vi "打开电脑摄像头获取图像.vi"() -> ()   [LabVIEW 2014]
uses:
  <vilib>/userdefined/High Color/IMAQdx.ctl
  <vilib>/vision/driver/NI_Vision_Acquisition_Software.lvlib
panel:
  out "Session Out":T1
  out "Image Out":T2(plugin-control)
  in  "停止":bool
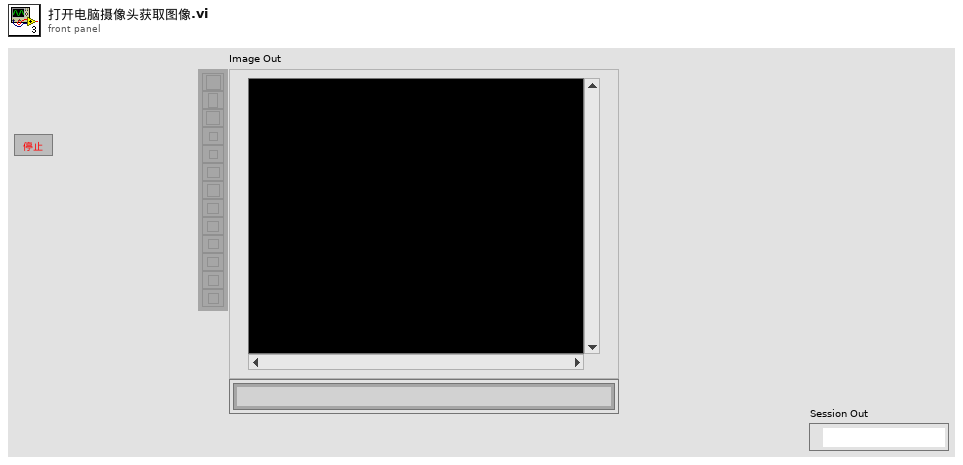
[diagram p1: front panel]
types:
  T1 = typedef "IMAQdx.ctl" = refnum<k21>
  T2 = typedef "IMAQ Image.ctl" = refnum<image>
  T3 = cluster{"Type":u32, "Version":u32, "Flags":u32, "SerialNumberHigh":u32, "SerialNumberLow":u32, "BusType":u32, "InterfaceName":string, "VendorName":string, "ModelName":string, "CameraFileName":string, "CameraAttributeURL":string}[]
  T4 = cluster{"Type":u32, "Version":u32, "Flags":u32, "SerialNumberHigh":u32, "SerialNumberLow":u32, "BusType":u32, "InterfaceName":string, "VendorName":string, "ModelName":string, "CameraFileName":string, "CameraAttributeURL":string}
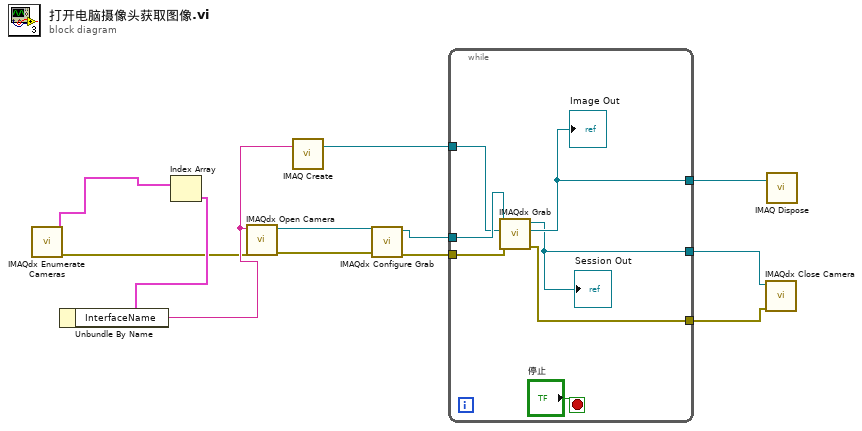
[diagram p0: block diagram]
diagram:
  n1 = call <vilib>:"IMAQdx Enumerate Cameras.vi"() -> ("error out"=w6:errorcluster, "Camera Information Array"=w12:T3)  [unwired: 10 in]
  n2 = Index Array(array=w12) -> (element=w11:T4)  [unwired: 1 in]
  n3 = Unbundle By Name(w11) -> ("InterfaceName"=w10:string)
  n4 = call <vilib>:"IMAQdx Open Camera.vi"("error in"=w6, "Session In"=w10) -> ("error out"=w5:errorcluster, "Session Out"=w9:T1)  [unwired: 8 in]
  n5 = call "IMAQ Create"("Image Name"=w10) -> ("New Image"=w8:T2)  [unwired: 4 in, 1 out]
  n6 = call <vilib>:"IMAQdx Configure Grab.vi"("error in"=w5, "Session In"=w9) -> ("error out"=w4:errorcluster, "Session Out"=w7:T1)  [unwired: 8 in]
  n7 = while {
    tunnel: w8 -> [w16]
    tunnel: w7 -> [w17]
    tunnel: w4 -> [w18]
    tunnel: [w15] -> w3
    tunnel: [w14] -> w2
    tunnel: [w13] -> w1
    stop <- "停止" stop-if-true
    n8 = call <vilib>:"IMAQdx Grab.vi"("error in"=w18, "Image In"=w16, "Session In"=w17) -> ("error out"=w13:errorcluster, "Image Out"=w15:T2, "Session Out"=w14:T1)  [unwired: 5 in, 1 out]
    "Image Out" <- w15
    "Session Out" <- w14
  }
  n9 = call <vilib>:"IMAQdx Close Camera.vi"("error in"=w1, "Session In"=w2) -> ()  [unwired: 9 in, 1 out]
  n10 = call "IMAQ Dispose"("Image"=w3) -> ()  [unwired: 5 in, 1 out]
